vi "write_to_file_appanding.vi"() -> ()   [LabVIEW 2017]
panel:
  in  "stop":bool
  in  "file path (use dialog)":path
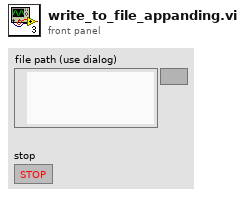
[diagram p1: front panel]
types:
  T1 = enum16{"open", "replace", "create", "open or create", "replace or create", "replace or create with confirmation"}
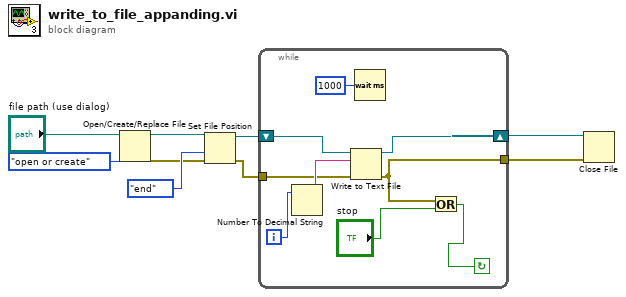
[diagram p0: block diagram]
diagram:
  n1 = Open/Create/Replace File(file path (use dialog)="file path (use dialog)", operation (0:open)=T1."open or create") -> (refnum out=w6:refnum<file>, error out=w1:errorcluster)  [unwired: 4 in, 1 out]
  n2 = Set File Position(refnum=w6, from (0:start)=enum16{"start", "end", "current"}."end", error in=w1) -> (refnum out=w5:refnum<file>, error out=w2:errorcluster)  [unwired: 1 in]
  n3 = while {
    shift-right: [w18] -> w7
    shift-left: w5 -> [w17]
    tunnel: [w11] -> w3
    tunnel: w2 -> [w10]
    i -> [w15]
    stop <- w12 continue-if-true
    n4 = Number To Decimal String(number=w15) -> (decimal integer string=w16:string)  [unwired: 1 in]
    n5 = Write to Text File(file (use dialog)=w17, text=w16, error in=w10) -> (refnum out=w18:refnum<file>, error out=w11:errorcluster)  [unwired: 1 in, 1 out]
    n6 = Wait (ms)(milliseconds to wait=u32 1000) -> ()  [unwired: 1 out]
    n7 = Or(x=w11, y="stop") -> (x .or. y?=w12:bool)
  }
  n8 = Close File(refnum=w7, error in=w3) -> ()  [unwired: 2 out]
